vi "Image_Save To Clipboard.vi"(7 "Image Ref":refnum<vi>, 8 "Error":errorcluster, 9 "Image Range":T1, 11 "Image":picture) -> (0 "Error Out":errorcluster)   [LabVIEW 2021]
uses:
  <vilib>/Utility/miscctls.llb/LVRectTypeDef.ctl
  <vilib>/Utility/miscctls.llb/LVBoundsTypeDef.ctl
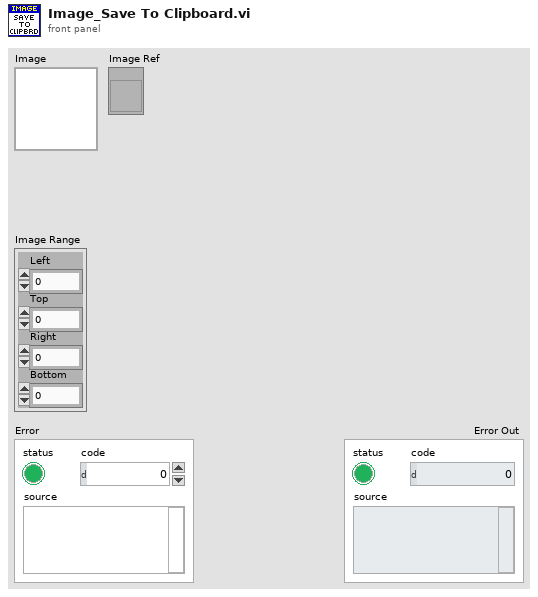
[diagram p1: front panel]
types:
  T1 = typedef "LVRectTypeDef.ctl" = cluster{"Left":i16, "Top":i16, "Right":i16, "Bottom":i16}
  T2 = typedef "LVBoundsTypeDef.ctl" = cluster{"Width":u32, "Height":u32}
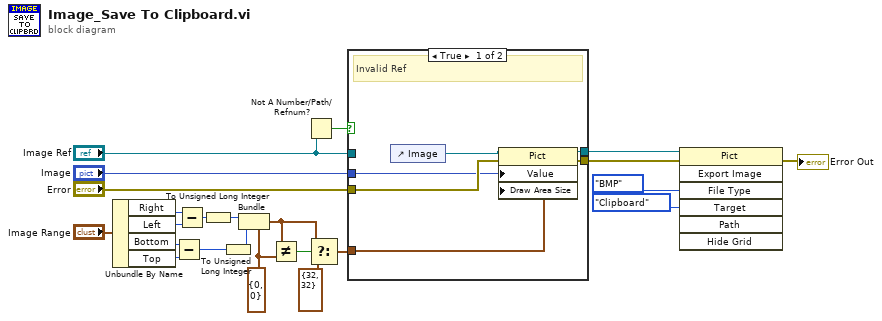
[diagram p0: block diagram]
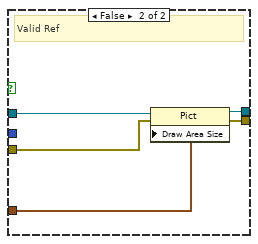
[diagram p2: hidden frame]
diagram:
  w5 = T2 {"Width"=0, "Height"=0} ("Area Size")
  n1 = Unbundle By Name("Image Range") -> ("Right"=w14:i16, "Left"=w13:i16, "Bottom"=w12:i16, "Top"=w11:i16)
  n2 = Subtract(x=w12, y=w11) -> (x-y=w10:i16)
  n3 = Subtract(x=w14, y=w13) -> (x-y=w9:i16)
  n4 = To Unsigned Long Integer(number=w9) -> (unsigned 32bit integer=w4:u32)
  n5 = To Unsigned Long Integer(number=w10) -> (unsigned 32bit integer=w3:u32)
  n6 = Bundle(cluster=w5, "Width"=w4, "Height"=w3) -> (w7:T2)
  n7 = Not Equal?(x=w7, y=w5) -> (x != y?=w8:bool)
  n8 = Not A Number/Path/Refnum?(number/path/refnum="Image Ref") -> (NaN/Path/Refnum?=w17:bool)
  n9 = Select(t=w7, s=w8, f=T2 {"Width"=32, "Height"=32} ("Area Size")) -> (s? t:f=w1:T2)
  n10 = case shown="True" w17 {
    tunnel: "Error" -> [w29 w34]
    tunnel: [w28 w33] -> w22
    tunnel: [w27 w32] -> w18
    tunnel: "Image" -> [w26 _]
    tunnel: "Image Ref" -> [_ w31]
    tunnel: w1 -> [w24 w30]
    frame True {
      # "Invalid Ref"
      n11 = control-ref of="Image"() -> (w25:refnum<vi>)
      n12 = property on="Property Node" class="Pict"(reference=w25, error in=w29, "Value"=w26, "Draw Area Size"=w24) -> (reference out=w28:refnum<vi>, error out=w27:errorcluster)
    }
    frame False {
      # "Valid Ref"
      n13 = property on="Property Node" class="Pict"(reference=w31, error in=w34, "Draw Area Size"=w30) -> (reference out=w33:refnum<vi>, error out=w32:errorcluster)
    }
  }
  n14 = invoke on="Invoke Node" class="Pict" method="Export Image"(reference=w22, error in=w18, "File Type"=enum32{"BMP", "EPS", "EMF", "PICT"}."BMP", "Target"=enum32{"File", "Clipboard"}."Clipboard") -> (error out=→"Error Out":errorcluster)  [unwired: 3 in, 6 out]
